vi "ReadSerial.vi"() -> ()   [LabVIEW 2020]
uses:
  <vilib>/Instr/_visa.llb/VISA Configure Serial Port (Instr).vi
panel:
  out "String":string
  in  "Numeric":u32
  in  "VISA resource name":refnum<visa-resource-name>
  in  "Stop Button":bool
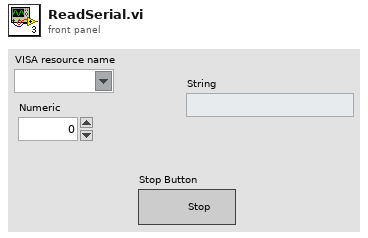
[diagram p1: front panel]
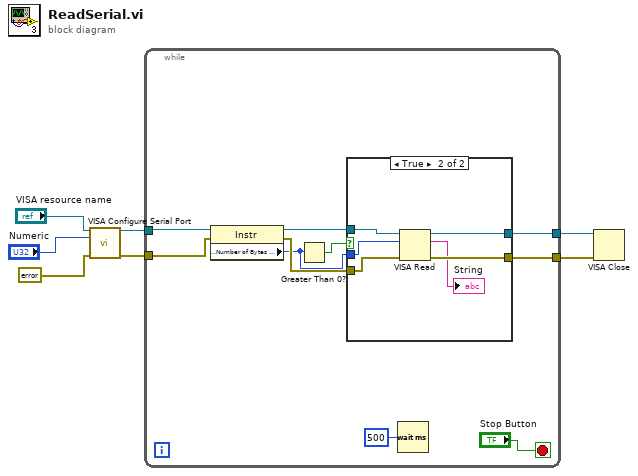
[diagram p0: block diagram]
diagram:
  n1 = call-poly "VISA Configure Serial Port"("VISA resource name"="VISA resource name", "baud rate (9600)"="Numeric", "error in (no error)"=errorcluster {"status"=FALSE, "code"=0, "source"=""} ("error constant")) -> ("VISA resource name out"=w4:refnum<visa-resource-name>, "error out"=w3:errorcluster)  [unwired: 11 in]
  n2 = while {
    tunnel: w4 -> [w15]
    tunnel: w3 -> [w14]
    tunnel: [w9] -> w2
    tunnel: [w8] -> w1
    stop <- "Stop Button" stop-if-true
    n3 = property class="Instr"(reference=w15, error in=w14) -> (reference out=w12:refnum<visa-resource-name>, error out=w11:errorcluster, "Serial Settings:Number of Bytes at Serial Port"=w10:u32)
    n4 = Greater Than 0?(x=w10) -> (x > 0?=w13:bool)
    n5 = case shown="True" w13 {
      tunnel: w12 -> [w19 w25]
      tunnel: w11 -> [w18 w24]
      tunnel: w10 -> [_ w23]
      tunnel: [w19 w22] -> w9
      tunnel: [w18 w21] -> w8
      frame False {
      }
      frame True {
        n6 = VISA Read(VISA resource name=w25, byte count=w23, error in (no error)=w24) -> (VISA resource name out=w22:refnum<visa-resource-name>, read buffer=→"String":string, error out=w21:errorcluster)  [unwired: 1 out]
      }
    }
    n7 = Wait (ms)(milliseconds to wait=u32 500) -> ()  [unwired: 1 out]
  }
  n8 = VISA Close(VISA resource name=w2, error in (no error)=w1) -> ()  [unwired: 1 out]
